vi "Assert String Not Starts With.vi"(5 "Prefix":string, 7 "Message (\"\")":string, 8 "error in (no error)":errorcluster, 10 "String":string) -> (0 "error out":errorcluster)   [LabVIEW 2017, in "Transparent Assertions.lvlib" / "Assertions.lvlib"]
doc: "Asserts that a string does not start with the expected prefix. Returns an error if the assertion fails, and optionally appends a custom message to the error."
uses:
  Assertions.lvlib
  Constraints/LogicalNot/LogicalNot.lvclass
  Constraints/String Starts With/String Starts With.lvclass
  C:/Users/pasca/Projects/Home/TransparentAssertions/src/Transparent Assertions/Constraints/Constraint/Constraint.lvclass
  Constraints/UnaryOperator/UnaryOperator.lvclass
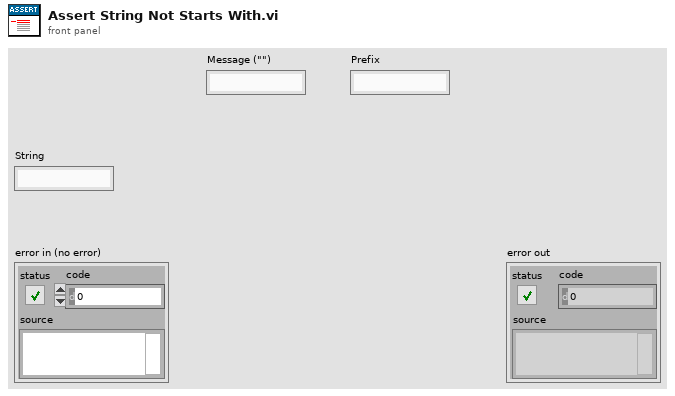
[diagram p1: front panel]
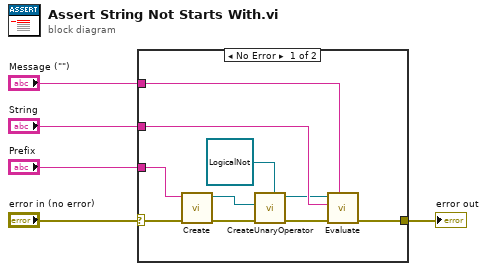
[diagram p0: block diagram]
diagram:
  n1 = case shown="No Error" "error in (no error)" {
    selector: "error in (no error)" -> [w11 w16]
    tunnel: "String" -> [w14 _]
    tunnel: [w13 w16] -> w4
    tunnel: "Message (\"\")" -> [w12 _]
    tunnel: "Prefix" -> [w10 _]
    frame No Error {
      n2 = call "Create.vi"("error in (no error)"=w11, "Prefix"=w10) -> ("error out"=w15:errorcluster, "String Starts With"=w8:refnum<class "String Starts With.lvclass">)  [unwired: 8 in]
      n3 = call-dynamic "CreateUnaryOperator.vi"("UnaryOperator In"=refnum<class "LogicalNot.lvclass"> refnum ("Transparent Assertions.lvlib:Constraints.lvlib:LogicalNot.lvclass"), "error in (no error)"=w15, "Constraint"=w8) -> ("error out"=w9:errorcluster, "UnaryOperator"=w7:refnum<class "UnaryOperator.lvclass">)  [unwired: 7 in]
      n4 = call-dynamic "Evaluate.vi"("Message (\"\")"=w12, "error in (no error)"=w9, "Actual"=w14, "Constraint in"=w7) -> ("error out"=w13:errorcluster)  [unwired: 6 in, 1 out]
    }
    frame Error {
    }
  }
  "error out" <- w4
